vi "Hella BLDC Pressure.vi"(8 "Error IN":errorcluster, 9 "Pressure":dbl, 10 "IGN":bool, 11 "Run?":bool) -> (0 "Error OUT":errorcluster)   [LabVIEW 2018]
uses:
  Type Defs/CAN Mode.ctl
panel:
  out "Actual Time (ms)":u32
  # "(100)"
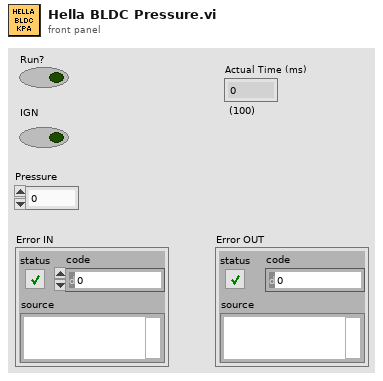
[diagram p1: front panel]
types:
  T1 = typedef "CAN Mode.ctl" = enum16{"Init", "Read", "Write", "Close"}
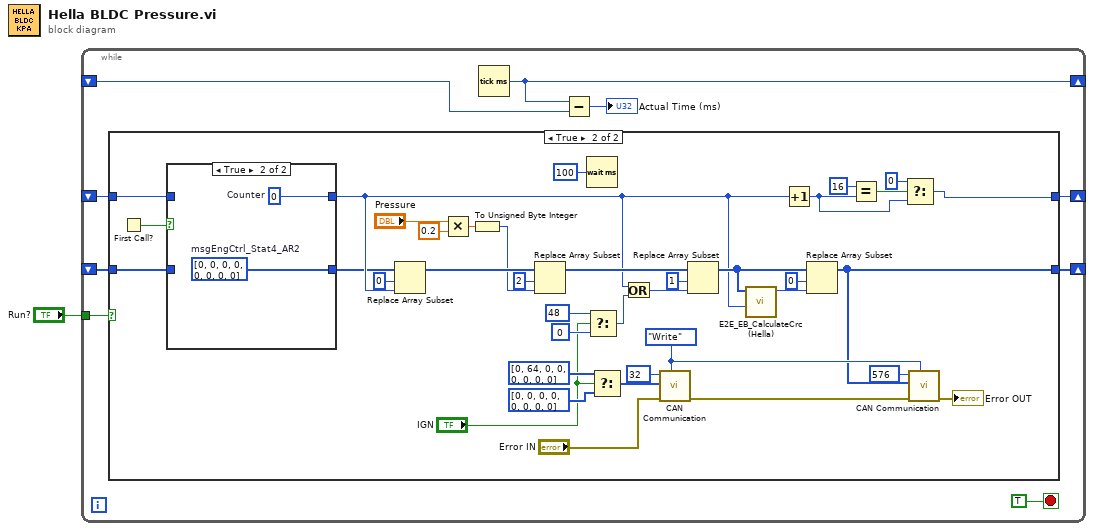
[diagram p0: block diagram]
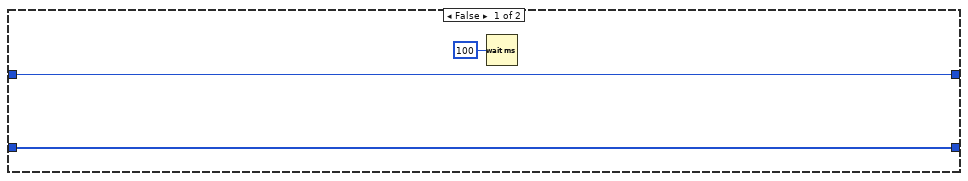
[diagram p2: hidden frame]
diagram:
  n1 = while {
    shift-right: [w10] -> _
    shift-left: _ -> [w8]
    shift-right: [w6] -> _
    shift-left: _ -> [w7]
    shift-right: [w2] -> _
    shift-left: _ -> [w3]
    tunnel: "Run?" -> [w5]
    stop <- TRUE stop-if-true
    n2 = case shown="True" w5 {
      tunnel: [w12 w35] -> w10
      tunnel: w8 -> [w12 w27]
      tunnel: w7 -> [w11 w26]
      tunnel: [w11 w15] -> w6
      frame False {
        n3 = Wait (ms)(milliseconds to wait=u32 100) -> ()  [unwired: 1 out]
      }
      frame True {
        w16 = CAN_Mode."Write" ("CAN Mode")
        n4 = First Call?() -> (First Call?: T/F=w23:bool)
        n5 = case shown="True" w23 {
          tunnel: w27 -> [w53 _]
          tunnel: w26 -> [w52 _]
          tunnel: [w53 w55] -> w25
          tunnel: [w52 w54] -> w24
          frame False {
          }
          frame True {
            w54 = u8[] [0, 0, 0, 0, 0, 0, 0, 0]  # msgEngCtrl_Stat4_AR2
            w55 = u8 0  # Counter
          }
        }
        n6 = Replace Array Subset(array=w24, new element=w25, index=0) -> (w48:u8[])
        n7 = Multiply(x="Pressure", y=0.2) -> (x*y=w47:dbl)
        n8 = To Unsigned Byte Integer(number=w47) -> (unsigned 8bit integer=w32:u8)
        n9 = Replace Array Subset(array=w48, new element=w32, index=2) -> (w28:u8[])
        n10 = Wait (ms)(milliseconds to wait=u32 100) -> ()  [unwired: 1 out]
        n11 = Select(t=u8 48, s="IGN", f=u8 0) -> (s? t:f=w42:u8)
        n12 = Select(t=u8[] [0, 64, 0, 0, 0, 0, 0, 0] ("Message"), s="IGN", f=u8[] [0, 0, 0, 0, 0, 0, 0, 0] ("Message")) -> (s? t:f=w18:u8[])
        n13 = Or(x=w25, y=w42) -> (x .or. y?=w41:u8)
        n14 = call "CAN Communication.vi"("CAN Mode"=w16, "Error IN"="Error IN", "Message"=w18, "Arbitration ID"=u32 32) -> ("Error OUT"=w20:errorcluster)  [unwired: 6 in, 1 out]
        n15 = Replace Array Subset(array=w28, new element=w41, index=1) -> (w29:u8[])
        n16 = call "E2E_EB_CalculateCrc (Hella).vi"("Counter"=w25, "Data"=w29) -> ("CrcValue"=w33:u8)  [unwired: 9 in]
        n17 = Increment(x=w25) -> (x+1=w37:u8)
        n18 = Replace Array Subset(array=w29, new element=w33, index=0) -> (w15:u8[])
        n19 = Equal?(x=u8 16, y=w37) -> (x = y?=w39:bool)
        n20 = Select(t=u8 0, s=w39, f=w37) -> (s? t:f=w35:u8)
        n21 = call "CAN Communication.vi"("CAN Mode"=w16, "Error IN"=w20, "Message"=w15, "Arbitration ID"=u32 576) -> ("Error OUT"=→"Error OUT":errorcluster)  [unwired: 6 in, 1 out]
      }
    }
    n22 = Tick Count (ms)() -> (millisecond timer value=w2:u32)
    n23 = Subtract(x=w2, y=w3) -> (x-y=→"Actual Time (ms)":u32)
  }
